vi "Set Source File.vi"(8 "error in (no error)":errorcluster, 10 "Source File":path, 11 "ImageLoad in":refnum<class "ImageLoad.lvclass">) -> (0 "error out":errorcluster, 3 "ImageLoad out":refnum<class "ImageLoad.lvclass">)   [LabVIEW 2015, in "ImageLoad.lvclass"]
uses:
  ImageLoad.lvclass
  ImageLoad.lvclass/ImageLoad.ctl
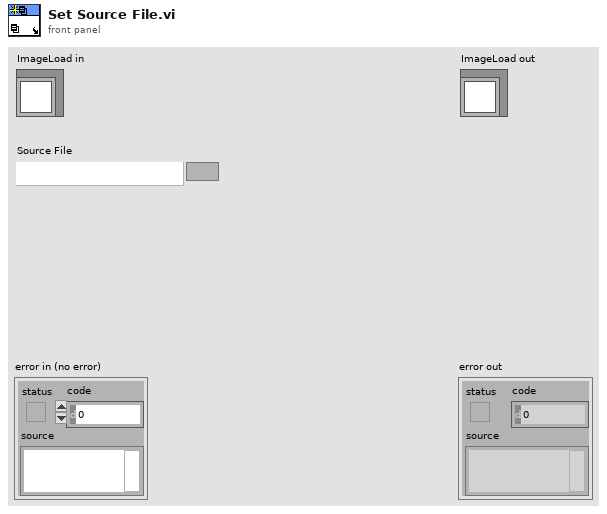
[diagram p1: front panel]
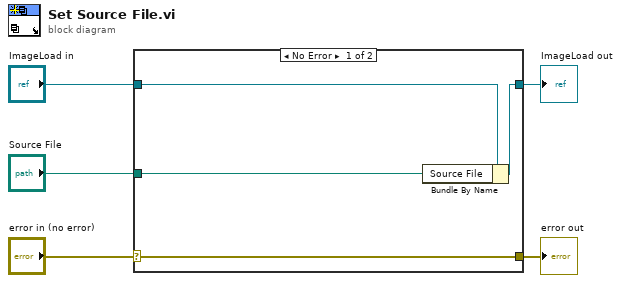
[diagram p0: block diagram]
diagram:
  n1 = case shown="No Error" "error in (no error)" {
    selector: "error in (no error)" -> [w9 w10]
    tunnel: [w9 w10] -> w4
    tunnel: [w7 w11] -> w2
    tunnel: "ImageLoad in" -> [w8 w11]
    tunnel: "Source File" -> [w6 _]
    frame No Error {
      n2 = Bundle By Name(cluster=w8, "Source File"=w6) -> (w7:refnum<class "ImageLoad.lvclass">)
    }
    frame Error {
    }
  }
  "error out" <- w4
  "ImageLoad out" <- w2
